vi "Conv Add Seconds to Date String.vi"(10 "Seconds Array":dbl[](array[numeric])=[1.0, 2.0, 3.0], 11 "Init Date String":string) -> (2 "Date Data":dbl[](array[numeric]), 3 "Time Array":string[](array[string]), 5 "Date Array":string[](array[string]))   [LabVIEW 2012]
panel:
  out "Time Stamp":timestamp
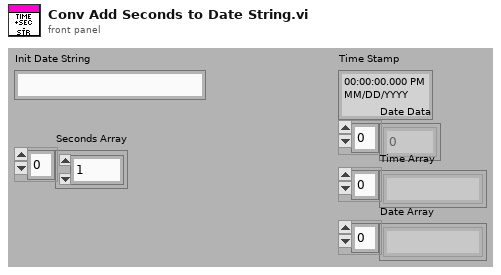
[diagram p1: front panel]
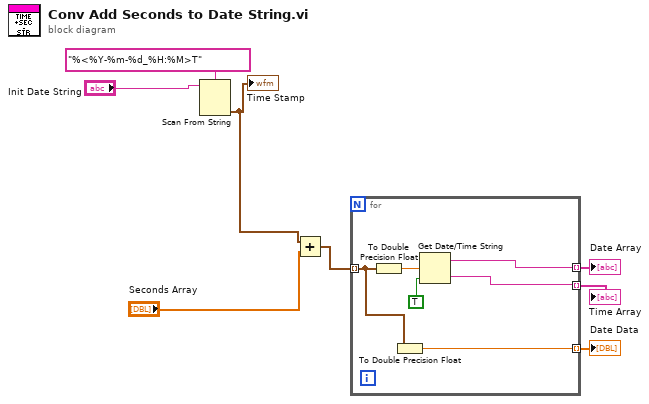
[diagram p0: block diagram]
diagram:
  n1 = Scan From String(format string="%<%Y-%m-%d_%H:%M>T" ("input string"), input string="Init Date String") -> (output 1=w5:timestamp)  [unwired: 3 in, 3 out]
  "Time Stamp" <- w5
  n2 = Add(x=w5, y="Seconds Array") -> (x+y=w4:timestamp[])
  n3 = for {
    tunnel: w4 -> [w12] mode=indexing
    tunnel: [w10] -> w3 mode=indexing
    tunnel: [w11] -> w2 mode=indexing
    tunnel: [w9] -> w1 mode=indexing
    n4 = To Double Precision Float(number=w12) -> (double precision float=w13:dbl)
    n5 = To Double Precision Float(number=w12) -> (double precision float=w11:dbl)
    n6 = Get Date/Time String(seconds (now)=w13, want seconds? (F)=TRUE) -> (date string=w10:string, time string=w9:string)  [unwired: 1 in]
  }
  "Date Array" <- w3
  "Date Data" <- w2
  "Time Array" <- w1
